vi "Get Entry by Index.vi"(8 "error in":errorcluster, 10 "Index":i32, 11 "Dictionary in":refnum<class "Dictionary.lvclass">) -> (0 "error out":errorcluster, 2 "Section":refnum<class "Section.lvclass">, 3 "Dictionary out":refnum<class "Dictionary.lvclass">)   [LabVIEW 2024, in "Electronic Datasheet.lvlib" / "Dictionary.lvclass"]
uses:
  Dictionary.lvclass
  OD Section/Section.lvclass
  Dictionary.lvclass/Dictionary.ctl
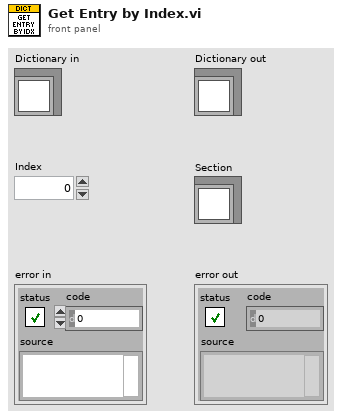
[diagram p1: front panel]
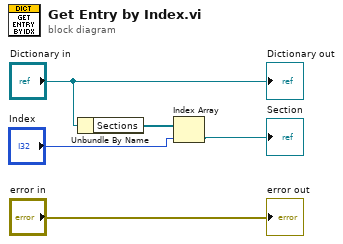
[diagram p0: block diagram]
diagram:
  n1 = Unbundle By Name("Dictionary in") -> ("Sections"=w3:refnum<class "Section.lvclass">[])
  n2 = Index Array(array=w3, index="Index") -> (element=→"Section":refnum<class "Section.lvclass">)
  "error out" <- "error in"
  "Dictionary out" <- "Dictionary in"
